vi "Generate Tabs.vi"(5 "indent":i32, 11 "error in (no error)":errorcluster) -> (4 "Tabs":string, 15 "error out":errorcluster)   [LabVIEW 2020, in "Variant JSON API.lvlib"]
doc: "Generates n number of tabs, where n is determined by the current Pretty Print Level."
uses:
  Variant JSON API.lvlib
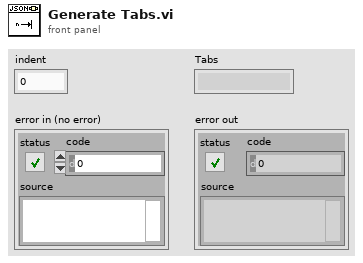
[diagram p1: front panel]
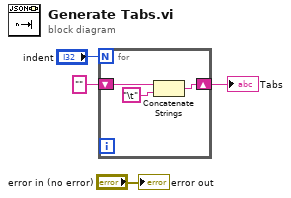
[diagram p0: block diagram]
diagram:
  n1 = for {
    N: "indent" -> [_]
    shift-right: [w5] -> w3
    shift-left: "" -> [w7]
    n2 = Concatenate Strings(w7, "\t") -> (w5:string)
  }
  "Tabs" <- w3
  "error out" <- "error in (no error)"
